vi "_getInfoForStaticGeneration.vi"(11 "Channels":T1[](array[typedef])) -> (1 "wfm info":cluster{i32, "variant":variant}[](array[cluster]), 3 "number of channels":i32)   [LabVIEW 2017]
uses:
  <vilib>/addons/InsightCM/Utilities/Analysis/Shared/controls/AnalysisSensorType.ctl
  <vilib>/addons/InsightCM/Utilities/Analysis/Shared/controls/AnalysisBandDomain.ctl
  <vilib>/addons/InsightCM/Utilities/Analysis/Shared/controls/AnalysisBandCalculation.ctl
  <vilib>/addons/InsightCM/Utilities/Analysis/Shared/controls/AnalysisBandAmplitudeScale.ctl
  <vilib>/addons/InsightCM/Utilities/Analysis/Shared/controls/AnalysisFeature.ctl
  <vilib>/addons/InsightCM/Utilities/Analysis/Shared/controls/AnalysisStaticChannel.ctl
  <vilib>/addons/InsightCM/Utilities/Analysis/Shared/controls/AnalysisCalculatedMeasurementType.ctl
  <vilib>/addons/InsightCM/MessageBus/Base/KeyValuePairs.ctl
  <vilib>/addons/InsightCM/MessageBus/Base/MetricInstance.ctl
  <vilib>/addons/InsightCM/MessageBus/Base/MetricConfiguration.ctl
  <vilib>/addons/InsightCM/MessageBus/Base/BlueRidgeChannel.ctl
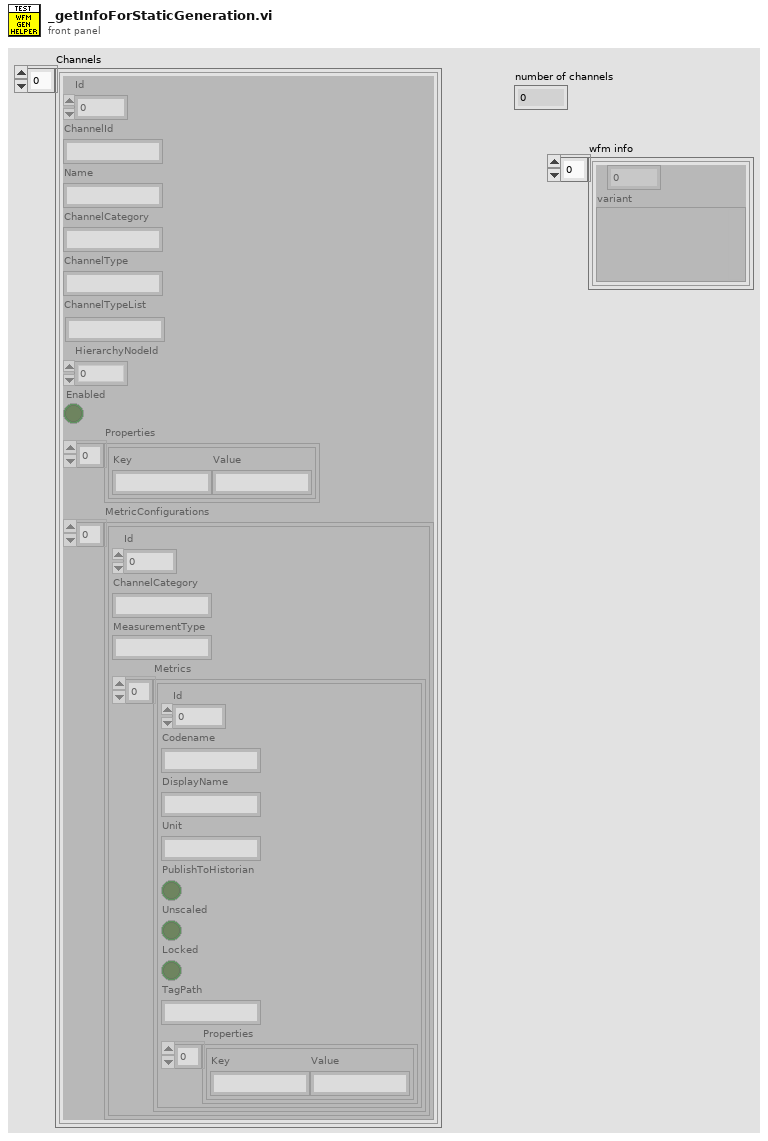
[diagram p1: front panel]
types:
  T1 = typedef "BlueRidgeChannel.ctl" = cluster{"Id":i32, "ChannelId":string, "Name":string, "ChannelCategory":string, "ChannelType":string, "ChannelTypeList":string, "HierarchyNodeId":i32, "Enabled":bool, "Properties":T2, "MetricConfigurations":T3[]}
  T2 = typedef "KeyValuePairs.ctl" = cluster{"Key":string, "Value":string}[]
  T3 = typedef "MetricConfiguration.ctl" = cluster{"Id":i32, "ChannelCategory":string, "MeasurementType":string, "Metrics":T4[]}
  T4 = typedef "MetricInstance.ctl" = cluster{"Id":i32, "Codename":string, "DisplayName":string, "Unit":string, "PublishToHistorian":bool, "Unscaled":bool, "Locked":bool, "TagPath":string, "Properties":T2}
  T5 = typedef "AnalysisStaticChannel.ctl" = cluster{"ChannelName":string, "Sensor Type":T6, "Features":T7[], "Properties":variant, "Data Valid":bool, "Calc Measurement Type":T11, "Acquisition Timestamp":timestamp}
  T6 = typedef "AnalysisSensorType.ctl" = enum16{"Accelerometer", "Velocity", "Displacement", "Tachometer", "Tempertature ", "dynamicVoltage", "Voltage", "Current", "Microphone", "Resistance", "Digital Input", "<Unknown>"}
  T7 = typedef "AnalysisFeature.ctl" = cluster{"Type":i32, "Code Name":string, "Unit":string, "Display Name":string, "Value":sgl, "Start":dbl, "Stop":dbl, "Band Domain":T8, "Band Calc":T9, "Amplitude Scale":T10, "Tag Path":string}
  T8 = typedef "AnalysisBandDomain.ctl" = enum16{"Frequency", "CPM", "Orders"}
  T9 = typedef "AnalysisBandCalculation.ctl" = enum16{"Total", "Max", "Phase"}
  T10 = typedef "AnalysisBandAmplitudeScale.ctl" = enum16{"rms", "peak", "pk-pk", "phase", "<none>"}
  T11 = typedef "AnalysisCalculatedMeasurementType.ctl" = enum16{"acceleration", "velocity", "displacement", "tachometer", "speed", "temperature", "voltage", "current", "resistance", "digitalInput", "<Unknown>"}
  T12 = typedef "AnalysisDynamicChannel.ctl" = cluster{"ChannelName":string, "Sensor Type":T6, "Conversion Op":T13, "Features":T7[], "Data":waveform(sgl), "Speed":sgl, "SP Index":i32, "Properties":variant, "Data Valid":bool, "Calc Measurement Type":T11}
  T13 = typedef "AnalysisConversionOp.ctl" = enum16{"none", "singleInt", "doubleInt", "singleDiff", "doubleDiff"}
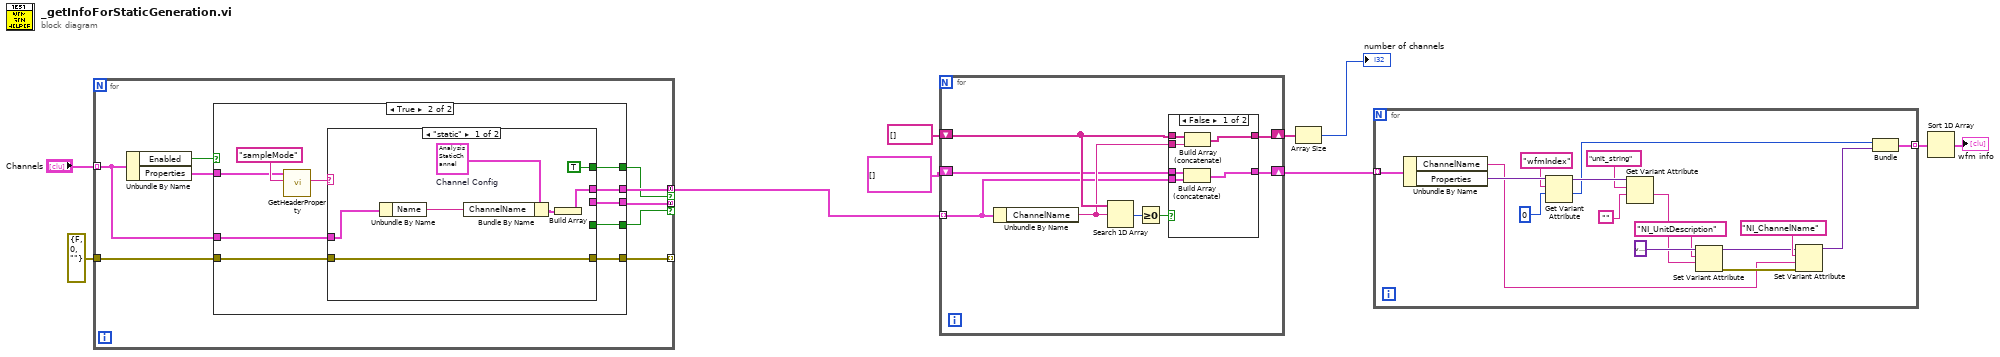
[diagram p0: block diagram]
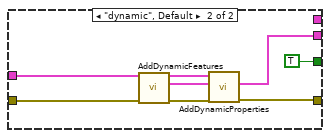
[diagram p3: hidden frame]
diagram:
  n1 = for {
    tunnel: "Channels" -> [w12] mode=indexing
    tunnel: [w17] -> _ mode=concatenating if=w15
    tunnel: errorcluster {"status"=FALSE, "code"=0, "source"=""} ("error IO") -> [w19]
    tunnel: [w18] -> _ mode=indexing
    tunnel: [w14] -> w1 mode=concatenating if=w13
    n2 = Unbundle By Name(w12) -> ("Enabled"=w16:bool, "Properties"=w11:T2)
    n3 = case shown="True" w16 {
      tunnel: w19 -> [w20 w26]
      tunnel: [w20 w27] -> w18
      tunnel: [_ w29] -> w17
      tunnel: [_ w30] -> w15
      tunnel: [_ w28] -> w13
      tunnel: [_ w25] -> w14
      tunnel: w12 -> [_ w22]
      tunnel: w11 -> [_ w21]
      frame False {
      }
      frame True {
        n4 = call <vilib>:"GetHeaderProperty.vi"("Key"="sampleMode", "Properties in"=w21) -> ("Value"=w23:string)  [unwired: 7 in, 2 out]
        n5 = case shown="\"static\"" w23 {
          tunnel: [_ TRUE] -> w30
          tunnel: [_ w41] -> w29
          tunnel: [TRUE _] -> w28
          tunnel: w26 -> [w35 w44]
          tunnel: [w35 w42] -> w27
          tunnel: [w34 _] -> w25
          tunnel: w22 -> [w32 w40]
          frame "static" {
            w36 = T5 {"ChannelName"="", "Sensor Type"=enum."Displacement", "Features"=[], "Properties"=variant, "Data Valid"=FALSE, "Calc Measurement Type"=enum."acceleration", "Acquisition Timestamp"=timestamp(0 s since 1904-01-01)}  # Channel Config
            n6 = Unbundle By Name(w32) -> ("Name"=w31:string)
            n7 = Bundle By Name(cluster=w36, "ChannelName"=w31) -> (w33:T5)
            n8 = Build Array(w33) -> (w34:T5[])
          }
          frame "dynamic", Default {
            n9 = call <vilib>:"AddDynamicFeatures.vi"("error in (no error)"=w44, "Asset Mgr Channel"=w40) -> ("error out"=w43:errorcluster, "Analysis Channels"=w38:T12[], "Asset Mgr Channel Out"=w39:T1)  [unwired: 7 in]
            n10 = call <vilib>:"AddDynamicProperties.vi"("error in (no error)"=w43, "Analysis Channels"=w38, "Asset Mgr Channel"=w39) -> ("error out"=w42:errorcluster, "Analysis Channels Out"=w41:T12[])  [unwired: 6 in, 1 out]
          }
        }
      }
    }
  }
  n11 = for {
    shift-right: [w50] -> w8
    shift-left: string[] [] -> [w51]
    tunnel: w1 -> [w48] mode=indexing
    shift-right: [w47] -> w7
    shift-left: T5[] [] -> [w46]
    n12 = Unbundle By Name(w48) -> ("ChannelName"=w49:string)
    n13 = Search 1D Array(1D array=w51, element=w49) -> (index of element=w52:i32)  [unwired: 1 in]
    n14 = Greater Or Equal To 0?(x=w52) -> (x >= 0?=w53:bool)
    n15 = case shown="False" w53 {
      tunnel: w51 -> [w59 w61]
      tunnel: [w58 w61] -> w50
      tunnel: w49 -> [w57 _]
      tunnel: w48 -> [w56 _]
      tunnel: [w55 w60] -> w47
      tunnel: w46 -> [w54 w60]
      frame False {
        n16 = Build Array (concatenate)(w54, w56) -> (w55:T5[])
        n17 = Build Array (concatenate)(w59, w57) -> (w58:string[])
      }
      frame True {
      }
    }
  }
  n18 = Array Size(array=w8) -> (size(s)=→"number of channels":i32)
  n19 = for {
    tunnel: w7 -> [w78] mode=indexing
    tunnel: [w62] -> w6 mode=indexing
    n20 = Unbundle By Name(w78) -> ("ChannelName"=w65:string, "Properties"=w77:variant)
    n21 = Get Variant Attribute(Variant=w77, name="wfmIndex", default value (empty Variant)=0) -> (duplicate Variant=w76:variant, value=w64:i32)  [unwired: 1 in, 2 out]
    n22 = Get Variant Attribute(Variant=w76, name="unit_string", default value (empty Variant)="") -> (value=w70:string)  [unwired: 1 in, 3 out]
    n23 = Set Variant Attribute(Variant=variant ("variant"), name="NI_UnitDescription", value=w70) -> (Variant out=w67:variant, error out=w66:errorcluster)  [unwired: 1 in, 1 out]
    n24 = Set Variant Attribute(Variant=w67, name="NI_ChannelName", value=w65, error in=w66) -> (Variant out=w63:variant)  [unwired: 2 out]
    n25 = Bundle(w64, "variant"=w63) -> (w62:cluster{i32, "variant":variant})  [unwired: 1 in]
  }
  n26 = Sort 1D Array(array=w6) -> (sorted array=→"wfm info":cluster{i32, "variant":variant}[])
